vi "OD Stats Formatter.vi"(5 "factor":dbl=1.0, 7 "Unit String":string=" ", 9 "OD History":T1(array[cluster])) -> (4 "Mean":dbl, 6 "Standard Deviation":dbl, 8 "Statistics String":string, 10 "Statistics String 2":string, 14 "Mean 2":dbl, 15 "Standard Deviation 2":dbl)   [LabVIEW 2009]
uses:
  <vilib>/Analysis/NI_AALBase.lvlib
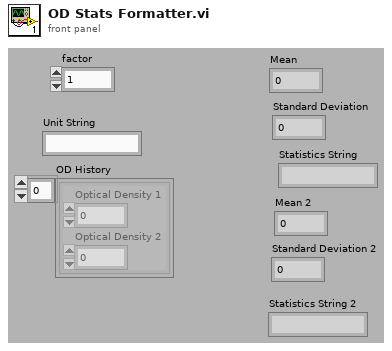
[diagram p1: front panel]
types:
  T1 = cluster{"Optical Density 1":dbl, "Optical Density 2":dbl}[]
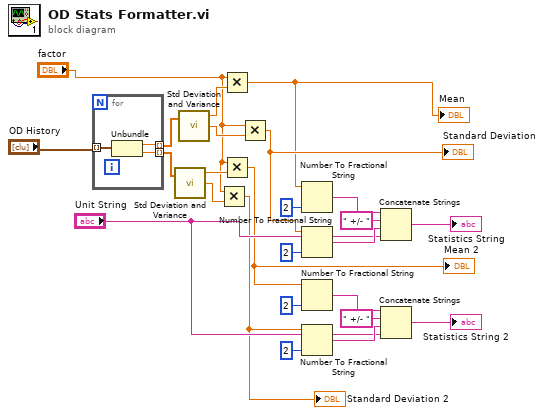
[diagram p0: block diagram]
diagram:
  n1 = for {
    tunnel: "OD History" -> [w27] mode=indexing
    tunnel: [w28] -> w15 mode=indexing
    tunnel: [w26] -> w13 mode=indexing
    n2 = Unbundle(w27) -> ("Optical Density 1"=w28:dbl, "Optical Density 2"=w26:dbl)
  }
  n3 = call <vilib>:"Std Deviation and Variance.vi"("X"=w13) -> ("mean"=w5:dbl, "standard deviation"=w2:dbl)  [unwired: 1 in, 1 out]
  n4 = call <vilib>:"Std Deviation and Variance.vi"("X"=w15) -> ("mean"=w16:dbl, "standard deviation"=w17:dbl)  [unwired: 1 in, 1 out]
  n5 = Multiply(x="factor", y=w2) -> (x*y=w1:dbl)
  "Standard Deviation 2" <- w1
  n6 = Multiply(x="factor", y=w16) -> (x*y=w18:dbl)
  "Mean" <- w18
  n7 = Multiply(x="factor", y=w5) -> (x*y=w4:dbl)
  "Mean 2" <- w4
  n8 = Multiply(x="factor", y=w17) -> (x*y=w20:dbl)
  "Standard Deviation" <- w20
  n9 = Number To Fractional String(number=w18, precision (6)=i16 2) -> (F-format string=w19:string)  [unwired: 2 out]
  n10 = Number To Fractional String(number=w20, precision (6)=i16 2) -> (F-format string=w21:string)  [unwired: 2 out]
  n11 = Number To Fractional String(number=w4, precision (6)=i16 2) -> (F-format string=w12:string)  [unwired: 2 out]
  n12 = Number To Fractional String(number=w1, precision (6)=i16 2) -> (F-format string=w11:string)  [unwired: 2 out]
  n13 = Concatenate Strings(w19, " +/- " ("string"), w21, "Unit String") -> (→"Statistics String":string)
  n14 = Concatenate Strings(w12, " +/- " ("string"), w11, "Unit String") -> (→"Statistics String 2":string)
